vi "Time-Delayed Send Message.vi"(6 "Message Priority (Normal)":T1=enum."Normal", 7 "# Copies (0 = infinite repeat)":u32, 8 "error in (no error)":errorcluster, 9 "Milliseconds To Wait":i32=1000, 10 "Message":refnum<class "Message.lvclass">, 11 "Message Enqueuer":refnum<class "Message Enqueuer.lvclass">) -> (0 "error out":errorcluster, 2 "Delivery Notifier":refnum<notifier>)   [LabVIEW 2013]
doc: "Waits for the specified amount of time and then sends a message to an actor a specified number of times."
uses:
  <vilib>/ActorFramework/Message Enqueuer/Message Enqueuer.lvclass
  <vilib>/ActorFramework/Message/Message.lvclass
  <vilib>/ActorFramework/Time-Delayed Send Message/Time-Delay Override Options.ctl
  <vilib>/ActorFramework/Message Enqueuer/Message Priority.ctl
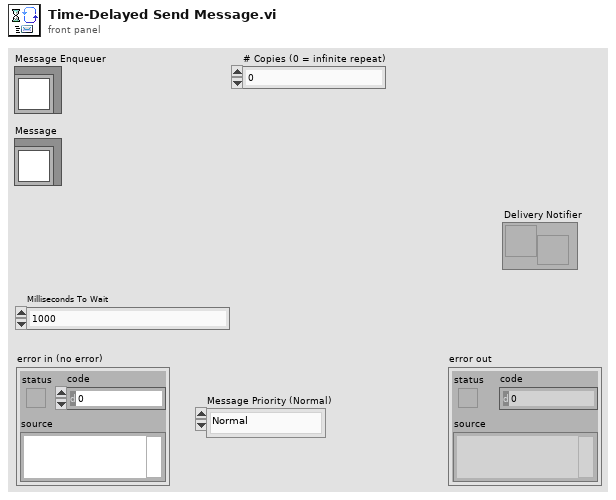
[diagram p1: front panel]
types:
  T1 = typedef "Actor Framework.lvlib/Message Enqueuer.lvclass/Message Priority.ctl" = enum16{"Low", "Normal", "High"}
  T2 = typedef "Time-Delay Override Options.ctl" = enum16{"Send next copy now", "Skip next scheduled copy", "Send next copy now and stop all further copies", "Stop all further copies"}
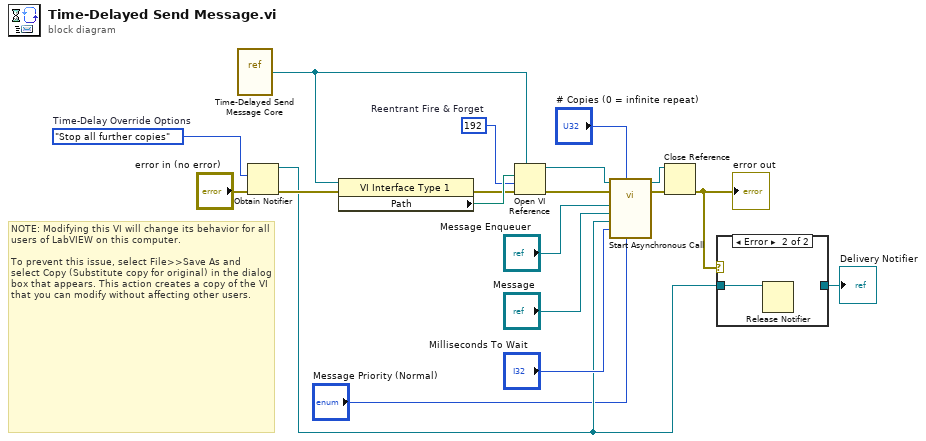
[diagram p0: block diagram]
diagram:
  w16 = 192  # Reentrant Fire & Forget
  w19 = Time-Delay_Override_Options."Stop all further copies"  # Time-Delay Override Options
  # "NOTE: Modifying this VI will change its behavior for all users of LabVIEW on this computer.\n\nTo prevent this issue, select File>>Save As and select Copy (Substitute copy for original) in the dialog box that appears. This action creates a copy of the VI that you can modify without affecting other users."
  n1 = vi-ref <vilib>:"Time-Delayed Send Message Core.vi"() -> (w3:refnum<vi>)
  n2 = Obtain Notifier(notification data type=w19, error in (no error)="error in (no error)") -> (notifier out=w2:refnum<notifier>, error out=w13:errorcluster)  [unwired: 2 in, 1 out]
  n3 = property class="VI Interface Type 1"(reference=w3, error in=w13) -> (error out=w14:errorcluster, "Path"=w17:path)  [unwired: 1 out]
  n4 = Open VI Reference(type specifier VI Refnum (for type only)=w3, vi path=w17, options=w16, error in (no error)=w14) -> (vi reference=w15:refnum<vi>, error out=w12:errorcluster)  [unwired: 2 in]
  n5 = call-by-ref "Start Asynchronous Call"(reference=w15, error in=w12, "Message Priority (Normal)"="Message Priority (Normal)", "How Many Copies (0 = infinite repeat)"="# Copies (0 = infinite repeat)", "Time To Wait"="Milliseconds To Wait", "Delivery Notifier"=w2, "Message"="Message", "Send Queue"="Message Enqueuer") -> (reference out=w10:refnum<vi>, error out=w11:errorcluster)  [unwired: 6 in]
  n6 = Close Reference(reference=w10, error in (no error)=w11) -> (error out=w9:errorcluster)
  "error out" <- w9
  n7 = case shown="Error" w9 {
    tunnel: [w20 _] -> w8
    tunnel: w2 -> [w20 w21]
    frame No Error {
    }
    frame Error {
      n8 = Release Notifier(notifier=w21) -> ()  [unwired: 2 in, 3 out]
    }
  }
  "Delivery Notifier" <- w8
